vi "CRYProject Editor PIC Load Dialog.vi"(8 "File Name":string, 10 "Sequence folder path":path) -> (0 "bResult":bool=TRUE, 2 "pPathFull":path)   [LabVIEW 2013]
panel:
  out "error out":errorcluster
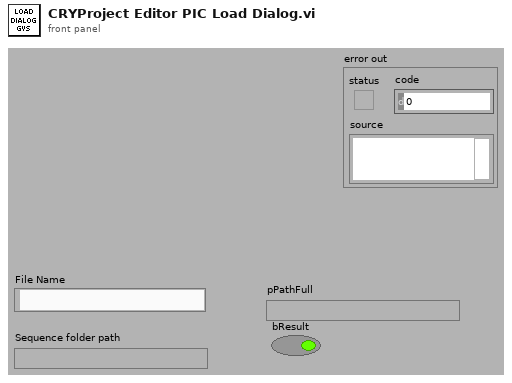
[diagram p1: front panel]
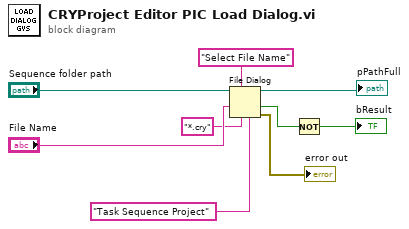
[diagram p0: block diagram]
diagram:
  n1 = File Dialog(4:"Task Sequence Project" ("pattern label"), 6:"*.cry" ("pattern (all files)"), 7:"Select File Name" ("prompt"), 9:"File Name", 11:"Sequence folder path") -> (0:→"error out":errorcluster, 1:w6:bool, 3:→"pPathFull":path)  [unwired: 1 in, 2 out]
  n2 = Not(x=w6) -> (.not. x?=→"bResult":bool)
